vi "Create.vi"(7 "mode settings":variant, 8 "error in":errorcluster, 9 "number of default channels":i32, 10 "channel settings":variant, 11 "mode in":refnum<class "Mode.lvclass">) -> (0 "error out":errorcluster, 1 "channels":refnum<class "Channel.lvclass">[](array[class]), 3 "mode out":refnum<class "Mode.lvclass">)   [LabVIEW 2017, in "Scan Engine Scripting.lvlib" / "Mode.lvclass"]
doc: "Creates a new instance of a mode."
uses:
  Mode.lvclass
  Channel Classes/Channel/Channel.lvclass
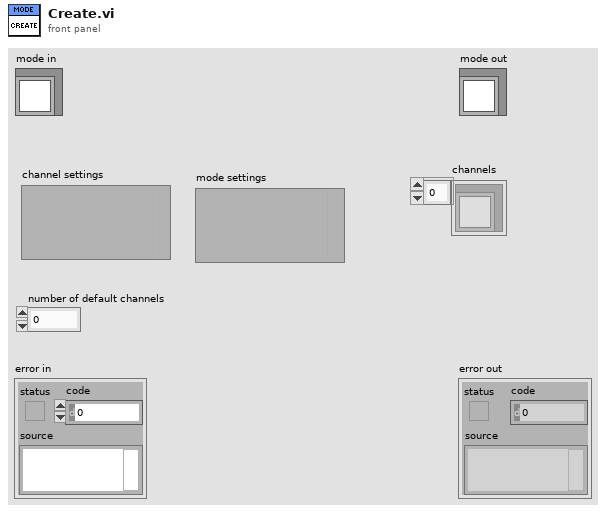
[diagram p1: front panel]
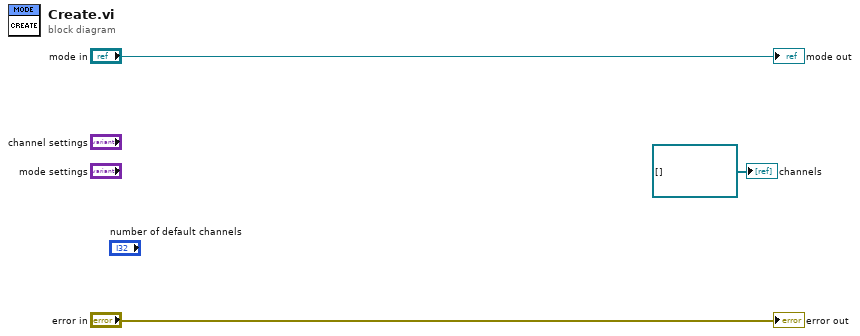
[diagram p0: block diagram]
diagram:
  "error out" <- "error in"
  "mode out" <- "mode in"
  "channels" <- refnum<class "Channel.lvclass">[] [] ("channels")
